vi "Read FW INI.vi"(8 "Error In":errorcluster, 11 "Firmware INI Path":path) -> (0 "Error Out":errorcluster, 2 "Firmware Config":T1, 3 "Duplicate Firmware INI Path":path)   [LabVIEW 2011, in "LVH-LINX.lvlib"]
uses:
  LVH-LINX.lvlib
  Type Defs/Device Firmware.ctl
  <vilib>/Utility/config.llb/Read Key (I32).vi
  <vilib>/Utility/config.llb/Read Key (String).vi
  <vilib>/Utility/config.llb/Read Key (Path).vi
  <vilib>/Utility/config.llb/NI_LVConfig.lvlib
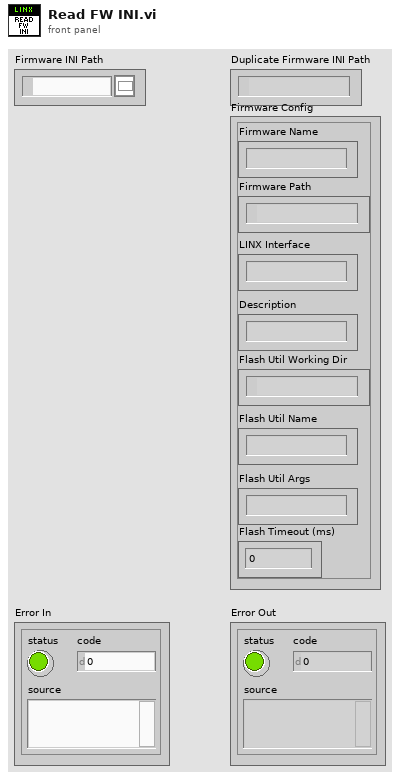
[diagram p1: front panel]
types:
  T1 = typedef "LVH-LINX.lvlib/Device Firmware.ctl" = cluster{"Firmware Name":string, "Firmware Path":path, "Description":string, "LINX Interface":string, "Flash Util Working Dir":path, "Flash Util Name":string, "Flash Util Args":string, "Flash Timeout (ms)":i32}
  T2 = typedef "NI_LVConfig.lvlib/Config Data RefNum.ctl" = refnum<k1>
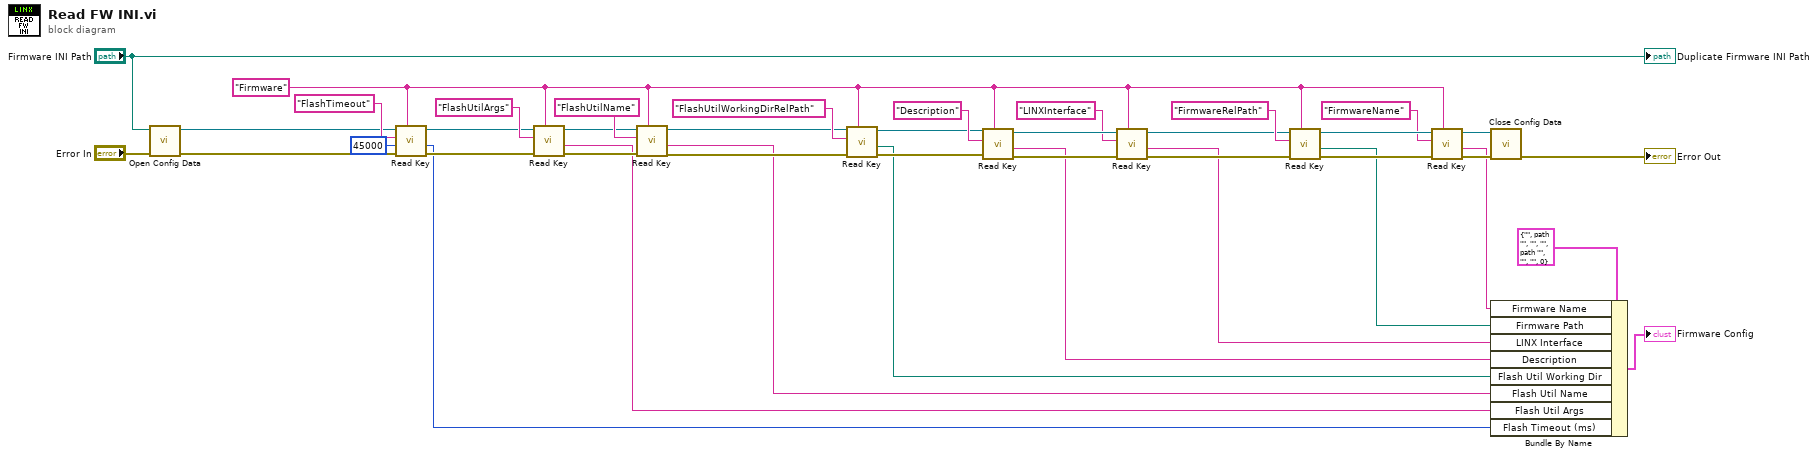
[diagram p0: block diagram]
diagram:
  w1 = "Firmware" ("key")
  n1 = call <vilib>:"Open Config Data.vi"("error in (no error)"="Error In", "configuration file path"="Firmware INI Path") -> ("error out"=w4:errorcluster, "refnum"=w5:T2)  [unwired: 7 in, 1 out]
  n2 = call-poly <vilib>:"Read Key.vi"("section"=w1, "error in (no error)"=w4, "default value"=45000, "key"="FlashTimeout", "refnum"=w5) -> ("error out"=w7:errorcluster, "value"=w2:i32, "refnum out"=w6:T2)  [unwired: 3 in, 1 out]
  n3 = call-poly <vilib>:"Read Key.vi"("section"=w1, "error in (no error)"=w7, "key"="FlashUtilArgs", "refnum"=w6) -> ("error out"=w15:errorcluster, "value"=w9:string, "refnum out"=w14:T2)  [unwired: 4 in, 1 out]
  n4 = call-poly <vilib>:"Read Key.vi"("section"=w1, "error in (no error)"=w15, "key"="FlashUtilName", "refnum"=w14) -> ("error out"=w16:errorcluster, "value"=w10:string, "refnum out"=w13:T2)  [unwired: 4 in, 1 out]
  n5 = call-poly <vilib>:"Read Key.vi"("section"=w1, "error in (no error)"=w16, "key"="FlashUtilWorkingDirRelPath", "refnum"=w13) -> ("error out"=w17:errorcluster, "value"=w11:path, "refnum out"=w12:T2)  [unwired: 4 in, 1 out]
  n6 = call-poly <vilib>:"Read Key.vi"("section"=w1, "error in (no error)"=w17, "key"="Description", "refnum"=w12) -> ("error out"=w32:errorcluster, "value"=w21:string, "refnum out"=w33:T2)  [unwired: 4 in, 1 out]
  n7 = call-poly <vilib>:"Read Key.vi"("section"=w1, "error in (no error)"=w32, "key"="LINXInterface", "refnum"=w33) -> ("error out"=w23:errorcluster, "value"=w22:string, "refnum out"=w24:T2)  [unwired: 4 in, 1 out]
  n8 = call-poly <vilib>:"Read Key.vi"("section"=w1, "error in (no error)"=w23, "key"="FirmwareRelPath", "refnum"=w24) -> ("error out"=w31:errorcluster, "value"=w26:path, "refnum out"=w34:T2)  [unwired: 4 in, 1 out]
  n9 = call-poly <vilib>:"Read Key.vi"("section"=w1, "error in (no error)"=w31, "key"="FirmwareName", "refnum"=w34) -> ("error out"=w36:errorcluster, "value"=w29:string, "refnum out"=w35:T2)  [unwired: 4 in, 1 out]
  n10 = call <vilib>:"Close Config Data.vi"("error in (no error)"=w36, "refnum"=w35) -> ("error out"=→"Error Out":errorcluster)  [unwired: 8 in, 1 out]
  n11 = Bundle By Name(cluster=T1 {"Firmware Name"="", "Firmware Path"=path "", "Description"="", "LINX Interface"="", "Flash Util Working Dir"=path "", "Flash Util Name"="", "Flash Util Args"="", "Flash Timeout (ms)"=0} ("Device Firmware"), "Firmware Name"=w29, "Firmware Path"=w26, "LINX Interface"=w22, "Description"=w21, "Flash Util Working Dir"=w11, "Flash Util Name"=w10, "Flash Util Args"=w9, "Flash Timeout (ms)"=w2) -> (→"Firmware Config":T1)
  "Duplicate Firmware INI Path" <- "Firmware INI Path"
